vi "SDSU_DacWithSwitches.vi"(0 "refnum":i32, 1 "register":bool, 3 "unit":string, 5 "first reg":i32, 9 "cmds":string[](array[string]), 11 "error in (no error)":errorcluster, 12 "sw args":string[](array[string]), 14 "swhitches":string[](array[string])) -> (4 "refnum out":i32, 6 "response":string, 15 "error out":errorcluster)   [LabVIEW 2016]
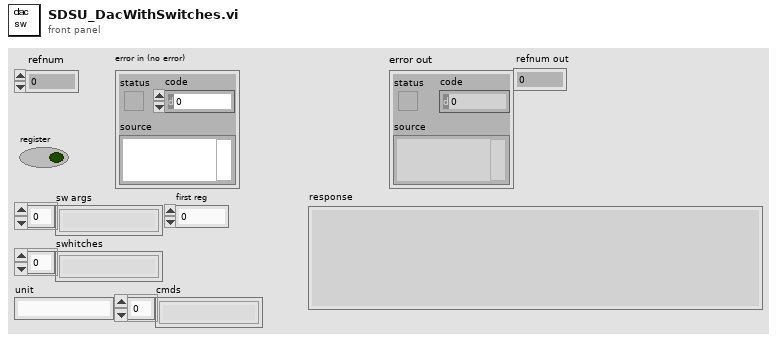
[diagram p1: front panel]
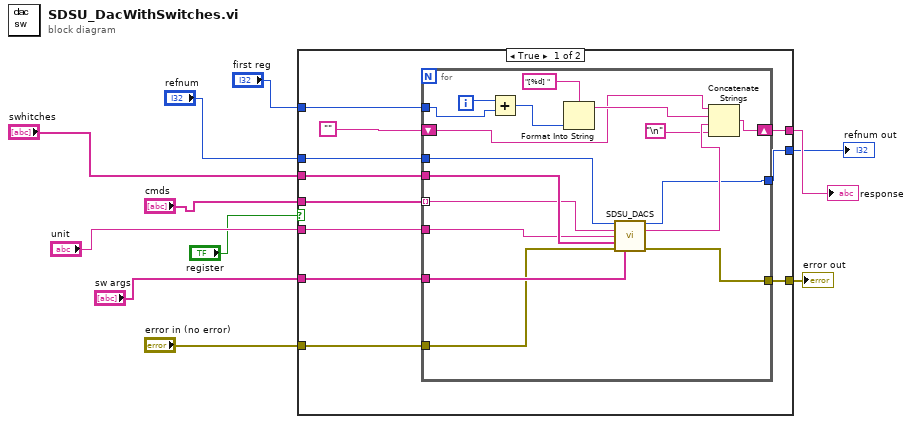
[diagram p0: block diagram]
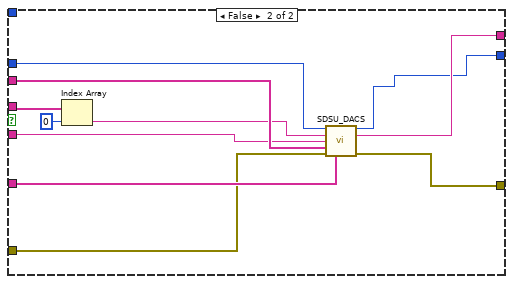
[diagram p2: hidden frame]
diagram:
  n1 = case shown="True" "register" {
    tunnel: [w22 w50] -> w11
    tunnel: "swhitches" -> [w21 w49]
    tunnel: "sw args" -> [w20 w48]
    tunnel: "unit" -> [w19 w47]
    tunnel: "cmds" -> [w12 w42]
    tunnel: [w18 w45] -> w10
    tunnel: "error in (no error)" -> [w16 w46]
    tunnel: "refnum" -> [w15 w44]
    tunnel: [w14 w43] -> w7
    tunnel: "first reg" -> [w13 _]
    frame True {
      n2 = for {
        tunnel: [w39] -> w22
        tunnel: w21 -> [w38]
        tunnel: w20 -> [w37]
        tunnel: w19 -> [w36]
        tunnel: w12 -> [w35] mode=indexing
        shift-right: [w33] -> w18
        shift-left: "" -> [w23]
        tunnel: w16 -> [w31]
        tunnel: w15 -> [w30]
        tunnel: [w29] -> w14
        tunnel: w13 -> [w27]
        i -> [w28]
        n3 = Add(x=w28, y=w27) -> (x+y=w26:i32)
        n4 = Format Into String(format string="[%d] ", w26) -> (resulting string=w24:string)  [unwired: 2 in, 1 out]
        n5 = call "SDSU_DACS.vi"("refnum"=w30, "Command"=w35, "physical unit"=w36, "swhitches"=w38, "error in (no error)"=w31, "switch arguments"=w37) -> ("refnum out"=w29:i32, "response"=w34:string, "error out"=w39:errorcluster)  [unwired: 7 out]
        n6 = Concatenate Strings(w23, w24, w34, "\n") -> (w33:string)
      }
    }
    frame False {
      n7 = Index Array(array=w42, index=0) -> (element=w40:string)
      n8 = call "SDSU_DACS.vi"("refnum"=w44, "Command"=w40, "physical unit"=w47, "swhitches"=w49, "error in (no error)"=w46, "switch arguments"=w48) -> ("refnum out"=w43:i32, "response"=w45:string, "error out"=w50:errorcluster)  [unwired: 7 out]
    }
  }
  "error out" <- w11
  "response" <- w10
  "refnum out" <- w7
